vi "2022-BeginLogic.vi"(1 "error in (no error)":errorcluster) -> (0 "error out":errorcluster)   [LabVIEW 2020]
uses:
  2023 Robot Global Data.vi
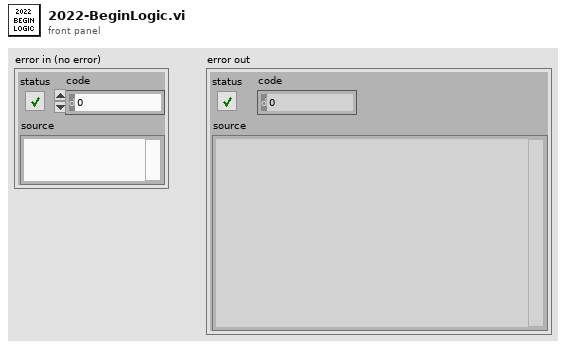
[diagram p1: front panel]
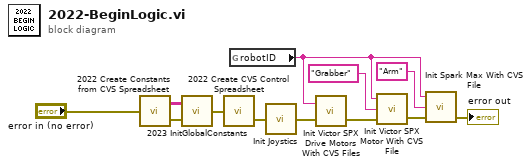
[diagram p0: block diagram]
diagram:
  n1 = call "2022 Create Constants from CVS Spreadsheet.vi"("error in"="error in (no error)") -> ("localConstantSpreadSheet"=w4:string[][], "error out"=w5:errorcluster)
  n2 = call "2023 InitGlobalConstants.vi"("error in (no error)"=w5, "localConstantSpreadSheet"=w4) -> ("error out"=w6:errorcluster)
  n3 = call "2022 Create CVS Control Spreadsheet.vi"("error in"=w6) -> ("error out"=w7:errorcluster)  [unwired: 1 out]
  n4 = global read "2023 Robot Global Data.vi" "robotID"() -> (w2:string)
  n5 = call "Init Joystics.vi"("error in"=w7) -> ("error out"=w8:errorcluster)
  n6 = call "Init Victor SPX Drive Motors With CVS Files.vi"("error in"=w8, "Robot ID"=w2) -> ("error out"=w9:errorcluster)  [unwired: 1 out]
  n7 = call "Init Victor SPX Motor With CVS File.vi"("error in"=w9, "Motor ID"="Grabber", "Robot ID"=w2) -> ("error out"=w10:errorcluster)  [unwired: 1 out]
  n8 = call "Init Spark Max With CVS File.vi"("error in"=w10, "Motor ID"="Arm", "Robot ID"=w2) -> ("error out"=→"error out":errorcluster)  [unwired: 1 in, 1 out]
